vi "GetSNLocation.vi"(0 "class data in":refnum<class "CMESAPI.lvclass">, 5 "serialNumber":string, 11 "error in (no error)":errorcluster) -> (4 "class data out":refnum<class "CMESAPI.lvclass">, 6 "GetSNLocation":string, 15 "error out":errorcluster)   [LabVIEW 2020, in "CMESAPI.lvlib" / "CMESAPI.lvclass"]
uses:
  CMESAPI.lvclass
  <vilib>/gpm_packages/@cs/event-logger/Source/Composed Log/Types/Log Level.ctl
  CMESAPI.lvclass/CMESAPI.ctl
  D:/Git/Labview-Libraries/Libraries/CMESAPI/CMESAPI_Fw4.0_1.9.2/CMESAPI.dll
  CMESAPI_Fw4.0_1.9.2/CMESAPI.dll
  <vilib>/gpm_packages/@cs/event-logger/Source/Composed Log/LoggerReference/LoggerReference.lvclass/LoggerReference.ctl
  <vilib>/gpm_packages/@cs/event-logger/Source/Composed Log/LoggerReference/Log.vi
  <vilib>/gpm_packages/@cs/event-logger/Source/Composed Log/LoggerReference/Get Valid Event Time.vi
  <vilib>/gpm_packages/@cs/event-logger/Source/Composed Log/LoggerReference/Remove Stale Logs.vi
  <vilib>/gpm_packages/@cs/event-logger/Source/Composed Log/LoggerReference/LoggerReference.lvclass
  <vilib>/gpm_packages/@cs/event-logger/Source/Composed Log/Composed Log.lvlib
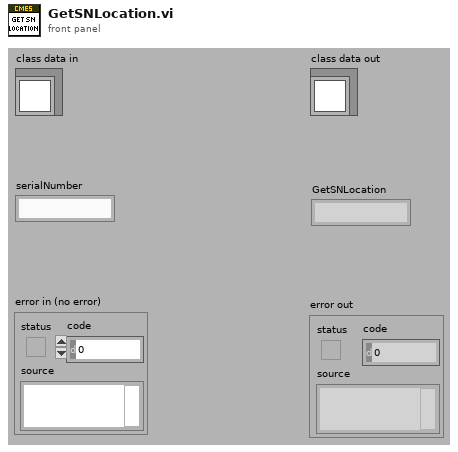
[diagram p1: front panel]
types:
  T1 = typedef "Composed Log.lvlib/Log Level.ctl" = enum16{"Debug", "Info", "Warning", "Error", "Critical"}
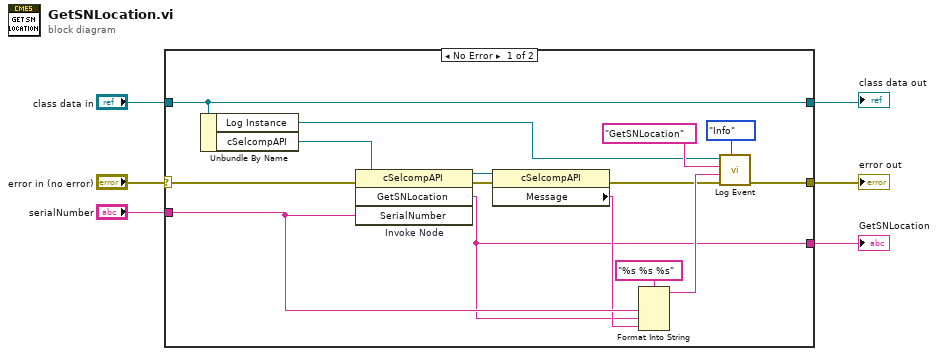
[diagram p0: block diagram]
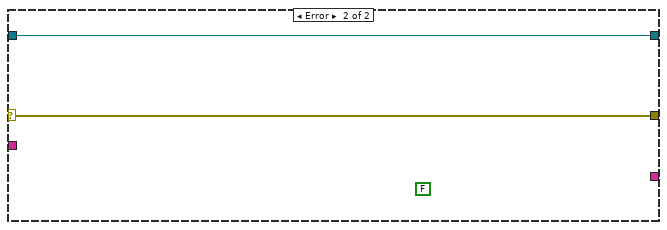
[diagram p2: hidden frame]
diagram:
  n1 = case shown="No Error" "error in (no error)" {
    selector: "error in (no error)" -> [w19 w23]
    tunnel: [w13 w23] -> w5
    tunnel: "class data in" -> [w21 w22]
    tunnel: [w21 w22] -> w3
    tunnel: "serialNumber" -> [w9 _]
    tunnel: [w7 _] -> w1
    frame No Error {
      n2 = Unbundle By Name(w21) -> ("Log Instance"=w12:refnum<class "LoggerReference.lvclass">, "cSelcompAPI"=w20:refnum<k24>)
      n3 = invoke on="Invoke Node" class="cSelcompAPI" method="GetSNLocation"(reference=w20, error in=w19, "SerialNumber"=w9) -> (reference out=w10:refnum<k24>, error out=w14:errorcluster, "GetSNLocation"=w7:string)  [unwired: 1 in, 1 out]
      n4 = property class="cSelcompAPI"(reference=w10, error in=w14) -> (error out=w11:errorcluster, "Message"=w8:string)  [unwired: 1 out]
      n5 = Format Into String(format string="%s %s %s", w9, w7, w8) -> (resulting string=w16:string)  [unwired: 2 in, 1 out]
      n6 = call <vilib>:"Log Event.vi"("Event Level"=Log_Level."Info", "error in (no error)"=w11, "Data To Log"=w16, "SourceID"="GetSNLocation", "Log Instance"=w12) -> ("error out"=w13:errorcluster)  [unwired: 5 in, 1 out]
    }
    frame Error {
      (unwired) FALSE ("CheckRouteForSerialNumber")
    }
  }
  "error out" <- w5
  "class data out" <- w3
  "GetSNLocation" <- w1
